vi "Init App.vi"(8 "error in (no error)":errorcluster, 11 "Post Analysis in":refnum<class "Post Analysis.lvclass">) -> (0 "error out":errorcluster, 3 "Post Analysis out":refnum<class "Post Analysis.lvclass">)   [LabVIEW 2023, in "Data Analysis.lvlib" / "Post Analysis.lvlib" / "Post Analysis.lvclass"]
uses:
  Post Analysis.lvclass
  Control/SideMenuBar.ctl
  Post Analysis.lvclass/Post Analysis.ctl
  Data Analysis.lvlib
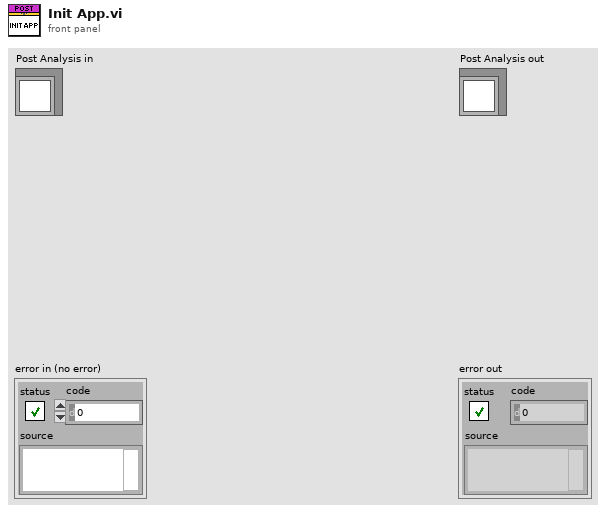
[diagram p1: front panel]
types:
  T1 = typedef "Data Analysis.lvlib/SideMenuBar.ctl" = enum32{"Test Info", "Error Log", "FE/FF Frame", "Signal Analysis", "Export Data", "Test Log Import/Export", "Info"}
  T2 = enum8{"Enabled", "Disabled", "Disabled and Grayed Out"}
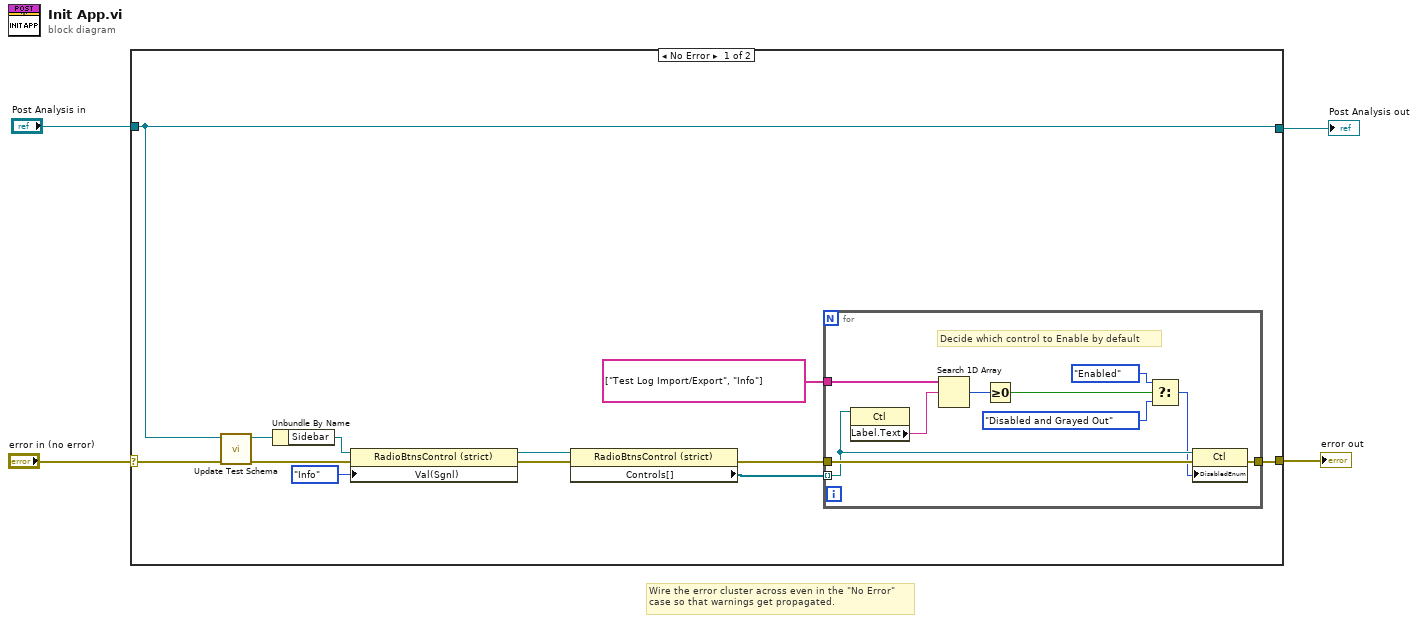
[diagram p0: block diagram]
diagram:
  # "Wire the error cluster across even in the \"No Error\"\ncase so that warnings get propagated."
  n1 = case shown="No Error" "error in (no error)" {
    selector: "error in (no error)" -> [w13 w28]
    tunnel: [w11 w27] -> w2
    tunnel: "Post Analysis in" -> [w11 w27]
    tunnel: [w14 w28] -> w1
    frame No Error {
      n2 = call "Update Test Schema.vi"("error in (no error)"=w13, "Post Analysis in"=w11) -> ("error out"=w12:errorcluster, "Post Analysis out"=w6:refnum<class "Post Analysis.lvclass">)  [unwired: 8 in]
      n3 = Unbundle By Name(w6) -> ("Sidebar"=w16:refnum<vi>)
      n4 = property class="RadioBtnsControl (strict)"(reference=w16, error in=w12, "Val(Sgnl)"=SideMenuBar."Info" ("Value (Signaling)")) -> (reference out=w9:refnum<vi>, error out=w8:errorcluster)
      n5 = property class="RadioBtnsControl (strict)"(reference=w9, error in=w8) -> (error out=w7:errorcluster, "Controls[]"=w15:refnum<vi>[])  [unwired: 1 out]
      n6 = for {
        tunnel: w15 -> [w24] mode=indexing
        tunnel: w7 -> [w26]
        tunnel: [w25] -> w14
        tunnel: string[] ["Test Log Import/Export", "Info"] -> [w19]
        # "Decide which control to Enable by default"
        n7 = property class="Ctl"(reference=w24) -> ("Label.Text"=w20:string)  [unwired: 1 in, 2 out]
        n8 = Search 1D Array(1D array=w19, element=w20) -> (index of element=w18:i32)  [unwired: 1 in]
        n9 = Greater Or Equal To 0?(x=w18) -> (x >= 0?=w17:bool)
        n10 = Select(t=T2."Enabled" ("Disabled"), s=w17, f=T2."Disabled and Grayed Out") -> (s? t:f=w21:T2)
        n11 = property class="Ctl"(reference=w24, error in=w26, "DisabledEnum"=w21) -> (error out=w25:errorcluster)  [unwired: 1 out]
      }
    }
    frame Error {
    }
  }
  "error out" <- w1
  "Post Analysis out" <- w2
